vi "Pneumatics_Command_Set_Tele.vi"(10 "Solenoid Command":T2, 11 "RT FIFO":u64) -> (3 "Cluster Out":T1)   [LabVIEW 2016]
uses:
  <userlib>/836-Libraries/Pneumatics/Support_Code/Pneumatics_Command.ctl
  <userlib>/836-Libraries/Pneumatics/Support_Code/Pneumatics_Notifier.ctl
  <userlib>/836-Libraries/Pneumatics/Support_Code/Pneumatics_Status.ctl
panel:
  in  "Pneumatics Notifier":T1
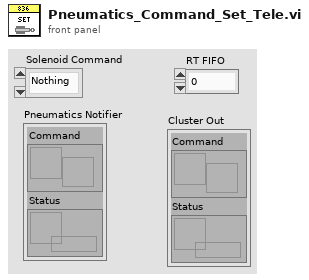
[diagram p1: front panel]
types:
  T1 = typedef "Pneumatics_Notifier.ctl" = cluster{"Command":refnum<notifier>, "Status":refnum<queue>}
  T2 = typedef "Pneumatics_Command.ctl" = enum16{"Nothing", "Forward", "Reverse", "Toggle"}
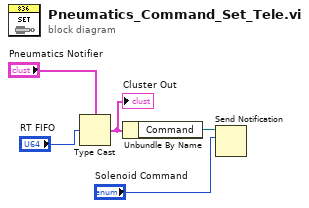
[diagram p0: block diagram]
diagram:
  n1 = Type Cast(type="Pneumatics Notifier", x="RT FIFO") -> (*(type *) &x=w3:T1)
  "Cluster Out" <- w3
  n2 = Unbundle By Name(w3) -> ("Command"=w5:refnum<notifier>)
  n3 = Send Notification(notification="Solenoid Command", notifier=w5) -> ()  [unwired: 1 in, 2 out]
